vi "IMAQReadMultiMetadata.vi"(8 "error in (no error)":errorcluster, 10 "Keys":string[](array[string]), 11 "Image In":T1) -> (0 "error out":errorcluster, 2 "Values":string[](array[string]), 3 "Image Out":T1)   [LabVIEW 2020]
uses:
  <vilib>/vision/Image Controls.llb/IMAQ Image.ctl
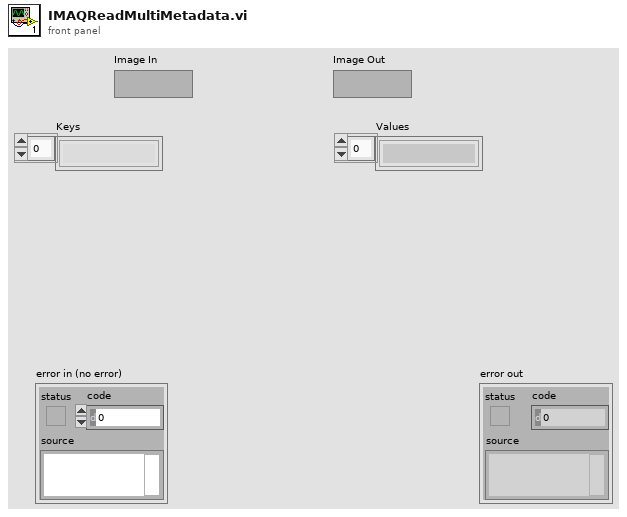
[diagram p1: front panel]
types:
  T1 = typedef "IMAQ Image.ctl" = refnum<image>
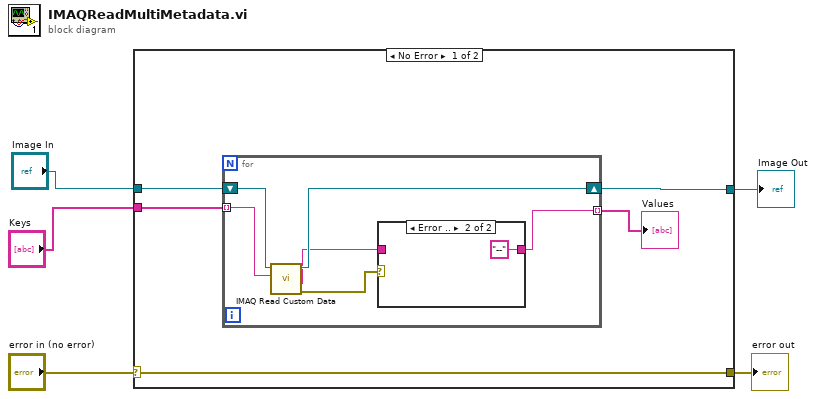
[diagram p0: block diagram]
diagram:
  n1 = case shown="No Error" "error in (no error)" {
    selector: "error in (no error)" -> [w10 w20]
    tunnel: [w10 w20] -> w4
    tunnel: "Image In" -> [w9 w19]
    tunnel: "Keys" -> [w8 _]
    tunnel: [w7 w19] -> w1
    frame No Error {
      n2 = for {
        tunnel: w8 -> [w14] mode=indexing
        shift-right: [w15] -> w7
        shift-left: w9 -> [w16]
        tunnel: [w11] -> w6 mode=indexing
        n3 = call "IMAQ Read Custom Data"("Key"=w14, "Image"=w16) -> ("error out"=w13:errorcluster, "Custom Data Out"=w12:string, "Image (duplicate)"=w15:T1)  [unwired: 7 in]
        n4 = case shown="Error .." w13 {
          tunnel: w12 -> [w17 _]
          tunnel: [w17 "--" ("Custom Data Out")] -> w11
          frame No Error {
          }
          frame Error {
          }
        }
      }
      "Values" <- w6
    }
    frame Error {
    }
  }
  "error out" <- w4
  "Image Out" <- w1
